vi "Main.vi"   [LabVIEW 2019, in "ModuleA.lvlib"]
uses:
  ModuleA.lvlib
  Communication/ABComm/Message1/Message1.lvclass
  Communication/ACComm/Message5/Message5.lvclass
  Utilities/FileUtilities/FileUtilities.lvlib
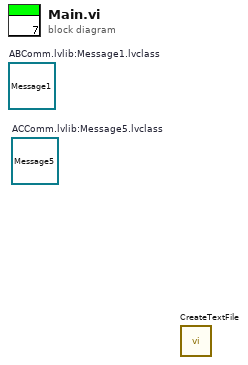
[diagram p0: block diagram]
diagram:
  (unwired) refnum<class "Message5.lvclass"> refnum  # ACComm.lvlib:Message5.lvclass
  (unwired) refnum<class "Message1.lvclass"> refnum  # ABComm.lvlib:Message1.lvclass
  n1 = call "CreateTextFile.vi"() -> ()  [unwired: 12 in]
